vi "penningeject.vi"() -> ()   [LabVIEW 2014, in "Panels.lvlib"]
uses:
  Panels.lvlib
  CSlibraries-extern/DimLVEvent/DimIndicators/DimIndicators.lvlib
  CSCore/CSSystem/CoreLib/CoreLib.lvlib
  CSlibraries/UtilityLib/UtilityLib.valueStatus.ctl
  CSlibraries/UtilityLib/UtilityLib.lvlib
  CSlibraries-extern/DimLVEvent/LVDimInterface/LVDimInterface.lvlib
  Instance           1 20Saved   penningeject .vi
  CSlibraries-extern/DimLVEvent/DimIndicators/DimIndicators.numericType.ctl
  CSlibraries-extern/DimLVEvent/DimIndicators/DimIndicators.numericArrayType.ctl
  CSlibraries-extern/DimLVEvent/DimIndicators/DimIndicators.anyType.ctl
panel:
  in  "EjPenDT2":bool
  out "EjPenDT2_Mon":dbl=inf format="%.4f"
  in  "EjPenDT6":bool
  out "EjPenDT6_Mon":dbl=inf format="%.4f"
  in  "SetFileLocation_Data":T1={"data"="NOLINK", "no link"=TRUE, "quality"=-1, "timeStamp"=0.0}
  in  "SetFileLocation":path=path "\\\\intranet\\Files/projects/lebit/Data Exchange/data/PenningEjectControl"
  in  "EjPenDT3":bool
  in  "EjPenDT4":bool
  in  "EjPenDT1":bool
  out "EjPenDT4_Mon":dbl=inf format="%.4f"
  out "EjPenDT3_Mon":dbl=inf format="%.4f"
  out "i ref out":refnum<vi>
  in  "Last Loaded File_Data":T1={"data"="NOLINK", "no link"=TRUE, "quality"=-1, "timeStamp"=0.0}
  out "FileUpToDate":bool=TRUE caption="Parameter Changed"
  in  "Close All Panels":bool
  in  "EjPenDT2_SetValueInfoData":T2={"data"=[], "no link"=TRUE, "quality"=-1, "timeStamp"=0.0}
  in  "EjPenDT3_SetValueInfoData":T2={"data"=[], "no link"=TRUE, "quality"=-1, "timeStamp"=0.0}
  in  "EjPenDT4_SetValueInfoData":T2={"data"=[], "no link"=TRUE, "quality"=-1, "timeStamp"=0.0}
  in  "EjPenDT6_SetValueInfoData":T2={"data"=[], "no link"=TRUE, "quality"=-1, "timeStamp"=0.0}
  in  "EjPenDT1_SetValueInfoData":T2={"data"=[], "no link"=TRUE, "quality"=-1, "timeStamp"=0.0}
  in  "EjPenDT1_SetData":T2={"data"=[], "no link"=TRUE, "quality"=-1, "timeStamp"=0.0}
  in  "EjPenDT6_SetData":T2={"data"=[], "no link"=TRUE, "quality"=-1, "timeStamp"=0.0}
  in  "EjPenDT4_SetData":T2={"data"=[], "no link"=TRUE, "quality"=-1, "timeStamp"=0.0}
  in  "EjPenDT3_SetData":T2={"data"=[], "no link"=TRUE, "quality"=-1, "timeStamp"=0.0}
  in  "EjPenDT2_SetData":T2={"data"=[], "no link"=TRUE, "quality"=-1, "timeStamp"=0.0}
  out "Last Loaded File":string
  in  "EjPenDT6_MonData":T3={"data"=inf, "no link"=TRUE, "quality"=-1, "timeStamp"=0.0}
  in  "EjPenDT4_MonData":T3={"data"=inf, "no link"=TRUE, "quality"=-1, "timeStamp"=0.0}
  in  "EjPenDT3_MonData":T3={"data"=inf, "no link"=TRUE, "quality"=-1, "timeStamp"=0.0}
  in  "EjPenDT2_MonData":T3={"data"=inf, "no link"=TRUE, "quality"=-1, "timeStamp"=0.0}
  in  "EjPenDT1_MonData":T3={"data"=inf, "no link"=TRUE, "quality"=-1, "timeStamp"=0.0}
  out "EjPenDT1_Mon":dbl=inf format="%.4f"
  out "EjPenDT5_Mon":dbl=inf format="%.4f"
  # "Parameter changed, data file is no longer up-to-date."
  # "EJPenDT5"
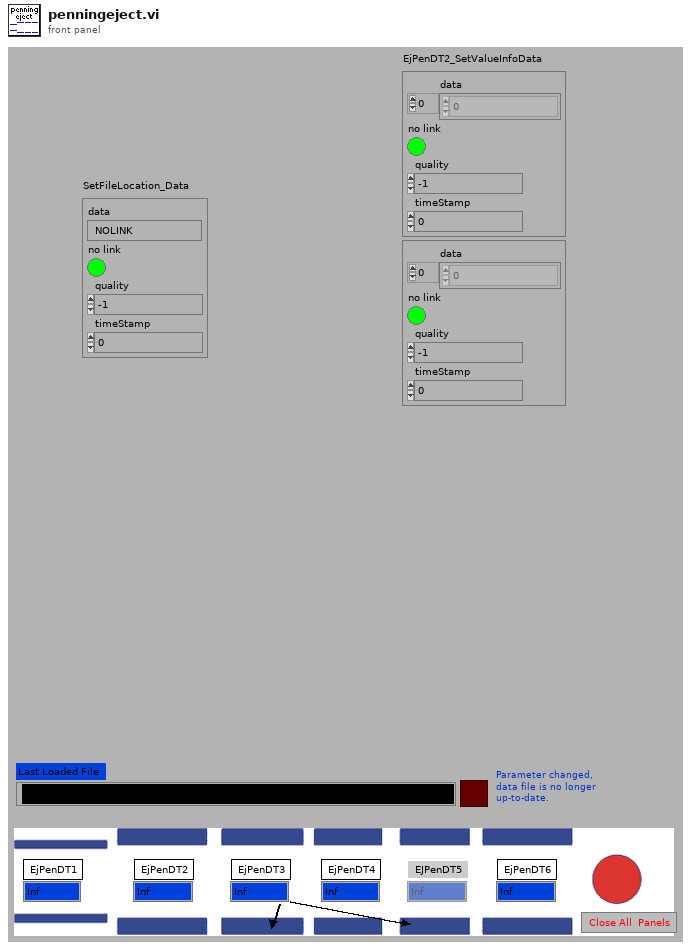
[diagram p1: front panel]
types:
  T1 = typedef "DimIndicators.lvlib/DimIndicators.anyType.ctl" = cluster{"data":string, "no link":bool, "quality":i32, "timeStamp":dbl}
  T2 = typedef "DimIndicators.lvlib/DimIndicators.numericArrayType.ctl" = cluster{"data":dbl[], "no link":bool, "quality":i32, "timeStamp":dbl}
  T3 = typedef "DimIndicators.lvlib/DimIndicators.numericType.ctl" = cluster{"data":dbl, "no link":bool, "quality":i32, "timeStamp":dbl}
  T4 = typedef "UtilityLib.lvlib/UtilityLib.valueStatus.ctl" = enum16{"no info available", "stand by/off", "on", "warning", "alarm/malfunction", "not implemented", "user action required", "important information", "system default", "control default", "indicator default", "button default"}
  T5 = cluster{"data":string, "no link":bool, "quality":i32, "timeStamp":dbl}
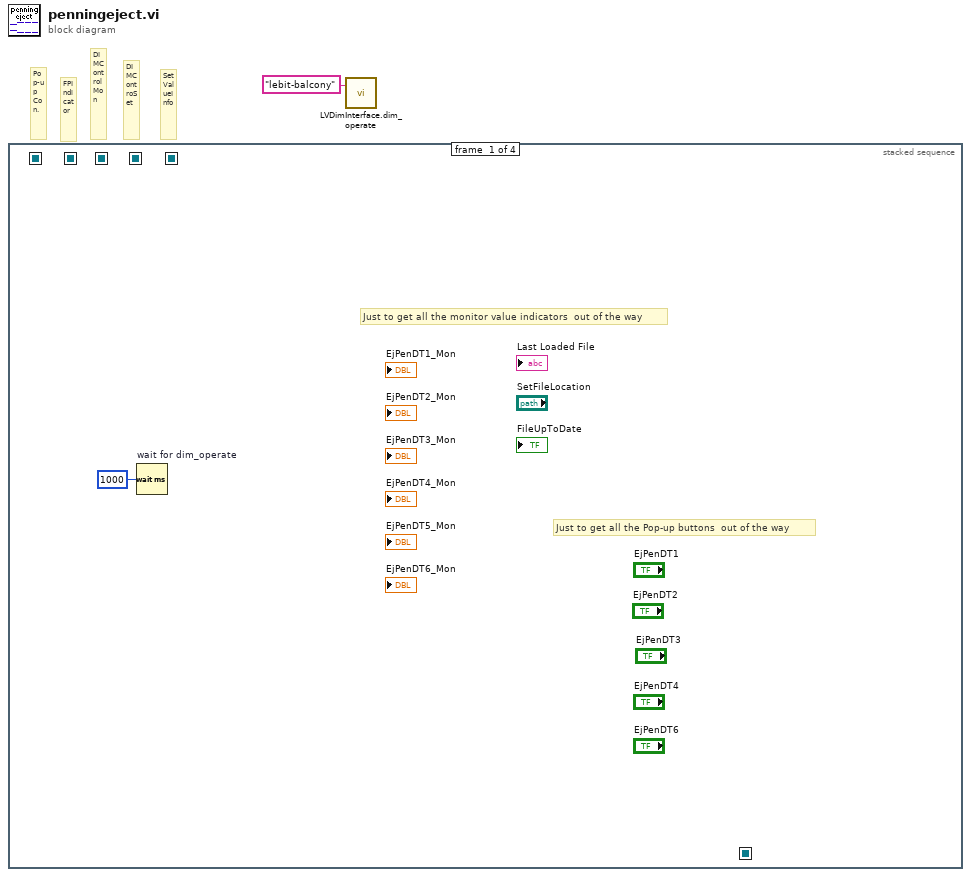
[diagram p0: block diagram]
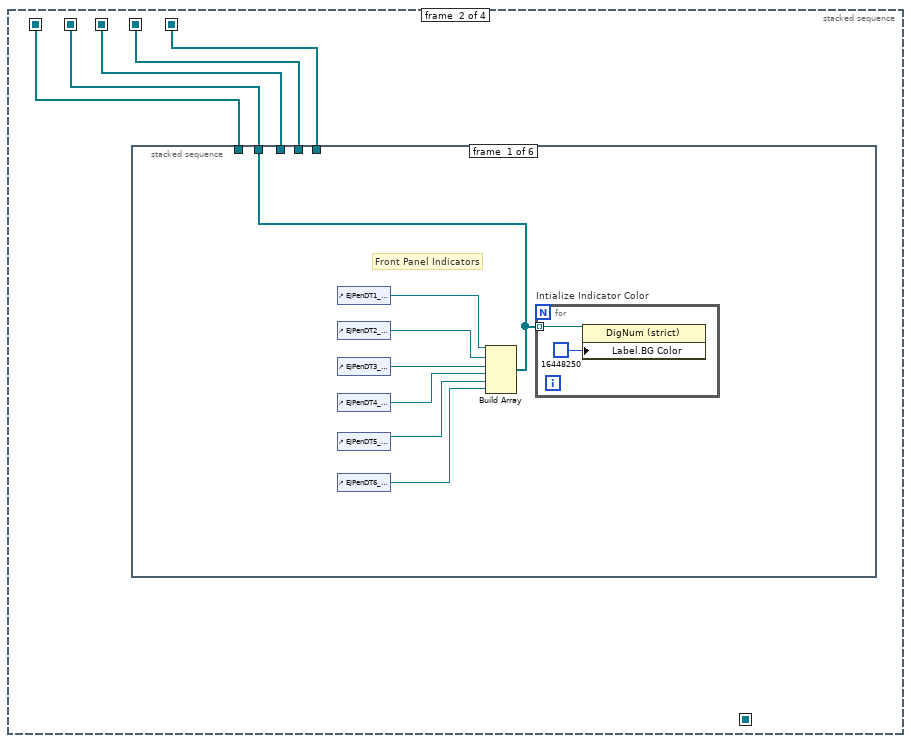
[diagram p2: hidden frame]
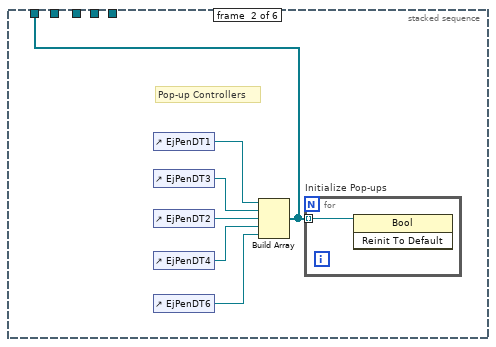
[diagram p3: hidden frame]
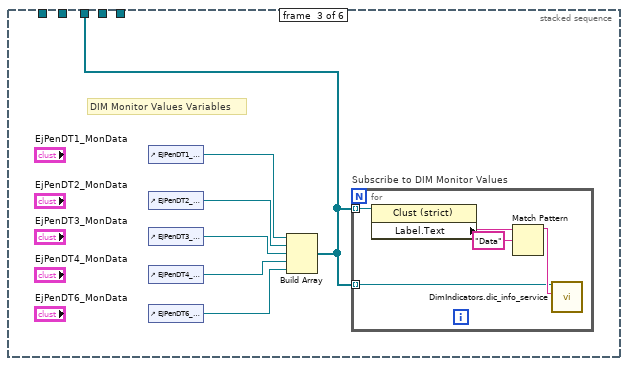
[diagram p4: hidden frame]
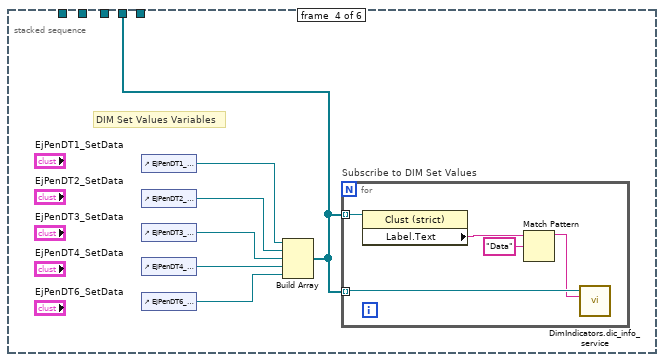
[diagram p5: hidden frame]
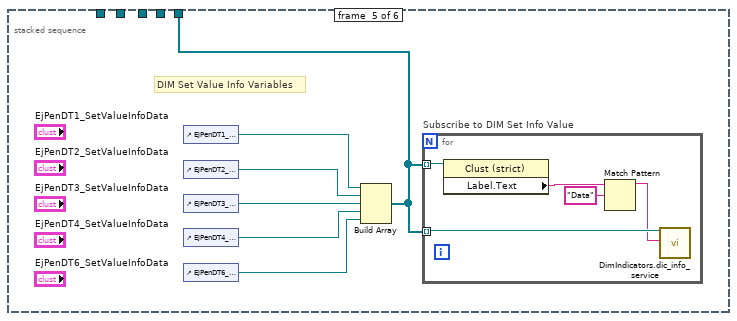
[diagram p6: hidden frame]
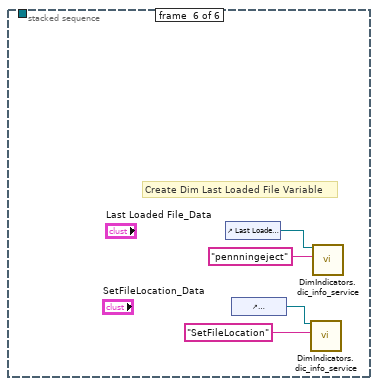
[diagram p7: hidden frame]
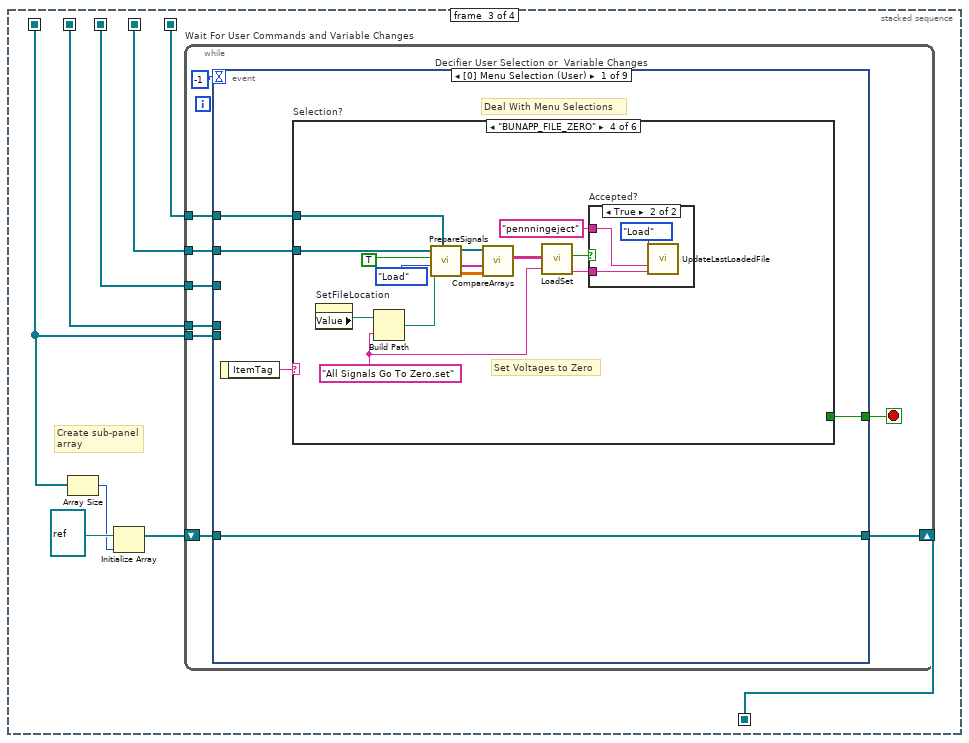
[diagram p8: hidden frame]
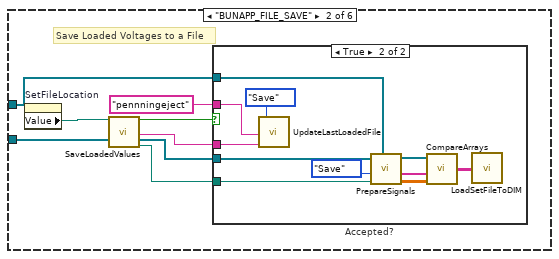
[diagram p10: hidden frame]
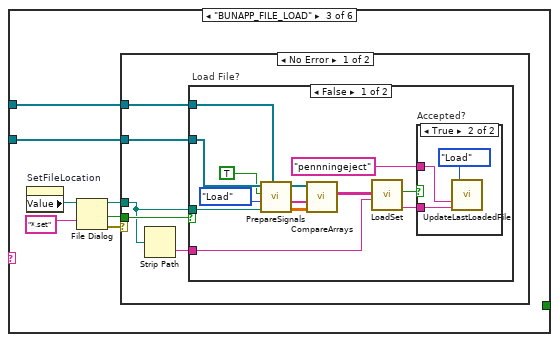
[diagram p12: hidden frame]
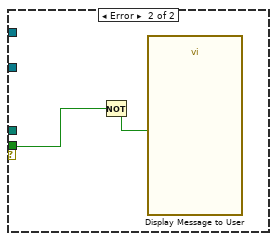
[diagram p15: hidden frame]
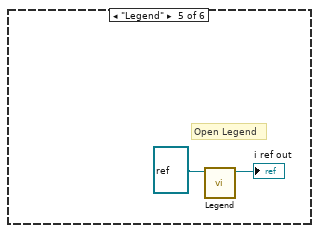
[diagram p17: hidden frame]
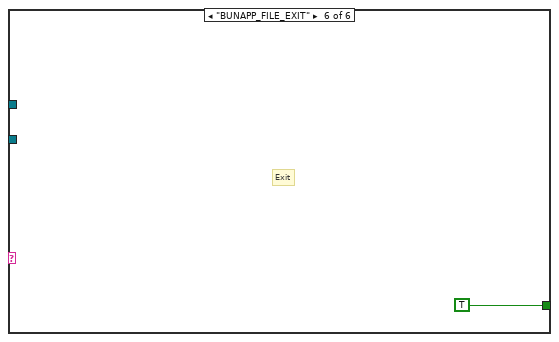
[diagram p18: hidden frame]
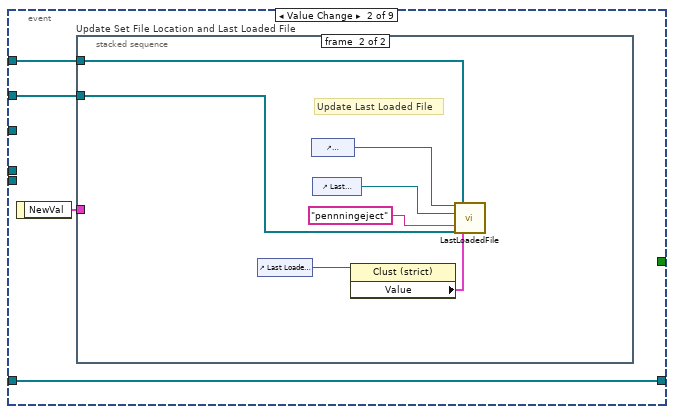
[diagram p19: hidden frame]
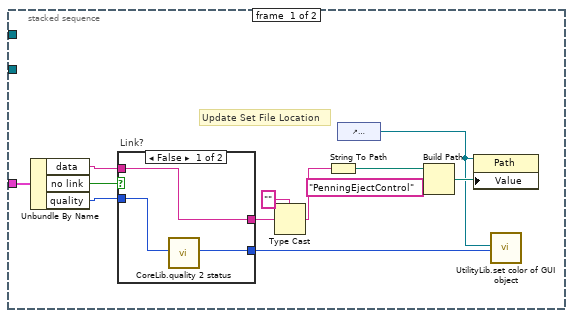
[diagram p20: hidden frame]
diagram:
  # "Pop-up Con."
  # "SetValueInfo"
  # "DIMControSet"
  # "DIMControlMon"
  # "FPIndicator"
  n1 = stacked-sequence {
    seq-local: [_ w7 _ _] -> [_ _ w66 _]
    seq-local: [_ w5 _ _] -> [_ _ w69 w265]
    seq-local: [_ _ w64 _] -> [_ _ _ w264]
    seq-local: [_ w4 _ _] -> [_ _ w63 w266]
    seq-local: [_ w3 _ _] -> [_ _ w62 w267]
    seq-local: [_ w6 _ _] -> [_ _ w61 _]
    frame #0 {
      # "Just to get all the Pop-up buttons  out of the way"
      # "Just to get all the monitor value indicators  out of the way"
      n2 = Wait (ms) "wait for dim_operate"(milliseconds to wait=u32 1000) -> ()  [unwired: 1 out]
    }
    frame #1 {
      # "Arrange references to all monitor-value related buttons into an array."
      n3 = stacked-sequence {
        tunnel: [w12 _ _ _ _ _] -> w7
        tunnel: [_ w19 _ _ _ _] -> w6
        tunnel: [_ _ w24 _ _ _] -> w5
        tunnel: [_ _ _ w35 _ _] -> w4
        tunnel: [_ _ _ _ w46 _] -> w3
        frame #0 {
          # "Front Panel Indicators"
          n4 = control-ref of="EjPenDT1_Mon"() -> (w11:refnum<vi>)
          n5 = control-ref of="EjPenDT2_Mon"() -> (w8:refnum<vi>)
          n6 = control-ref of="EjPenDT3_Mon"() -> (w10:refnum<vi>)
          n7 = control-ref of="EjPenDT4_Mon"() -> (w13:refnum<vi>)
          n8 = control-ref of="EjPenDT5_Mon"() -> (w14:refnum<vi>)
          n9 = control-ref of="EjPenDT6_Mon"() -> (w9:refnum<vi>)
          n10 = Build Array(w11, w8, w10, w13, w14, w9) -> (w12:refnum<vi>[])
          n11 = for "Intialize Indicator Color" {
            tunnel: w12 -> [w16] mode=indexing
            n12 = property class="DigNum (strict)"(reference=w16, "Label.BG Color"=u32 16448250 ("Color Box")) -> ()  [unwired: 1 in, 2 out]
          }
        }
        frame #1 {
          # "Pop-up Controllers"
          n13 = control-ref of="EjPenDT1"() -> (w22:refnum<vi>)
          n14 = control-ref of="EjPenDT3"() -> (w21:refnum<vi>)
          n15 = control-ref of="EjPenDT2"() -> (w18:refnum<vi>)
          n16 = control-ref of="EjPenDT4"() -> (w20:refnum<vi>)
          n17 = control-ref of="EjPenDT6"() -> (w17:refnum<vi>)
          n18 = Build Array(w22, w21, w18, w20, w17) -> (w19:refnum<vi>[])
          n19 = for "Initialize Pop-ups" {
            tunnel: w19 -> [w23] mode=indexing
            n20 = invoke class="Bool" method="Reinit To Default"(reference=w23) -> ()  [unwired: 2 in, 3 out]
          }
        }
        frame #2 {
          # "DIM Monitor Values Variables"
          n21 = control-ref of="EjPenDT1_MonData"() -> (w29:refnum<vi>)
          n22 = control-ref of="EjPenDT2_MonData"() -> (w28:refnum<vi>)
          n23 = control-ref of="EjPenDT3_MonData"() -> (w27:refnum<vi>)
          n24 = control-ref of="EjPenDT4_MonData"() -> (w26:refnum<vi>)
          n25 = control-ref of="EjPenDT6_MonData"() -> (w25:refnum<vi>)
          n26 = Build Array(w29, w28, w27, w26, w25) -> (w24:refnum<vi>[])
          n27 = for "Subscribe to DIM Monitor Values" {
            tunnel: w24 -> [w31] mode=indexing
            tunnel: w24 -> [w30] mode=indexing
            n28 = property class="Clust (strict)"(reference=w30) -> ("Label.Text"=w33:string)  [unwired: 1 in, 2 out]
            n29 = Match Pattern(string=w33, regular expression="Data") -> (before substring=w32:string)  [unwired: 1 in, 3 out]
            n30 = call "DimIndicators.dic_info_service.vi"("controlRef"=w31, "serviceName"=w32) -> ()  [unwired: 16 in, 2 out]
          }
        }
        frame #3 {
          # "DIM Set Values Variables"
          n31 = control-ref of="EjPenDT1_SetData"() -> (w40:refnum<vi>)
          n32 = control-ref of="EjPenDT2_SetData"() -> (w39:refnum<vi>)
          n33 = control-ref of="EjPenDT3_SetData"() -> (w38:refnum<vi>)
          n34 = control-ref of="EjPenDT4_SetData"() -> (w37:refnum<vi>)
          n35 = control-ref of="EjPenDT6_SetData"() -> (w36:refnum<vi>)
          n36 = Build Array(w40, w39, w38, w37, w36) -> (w35:refnum<vi>[])
          n37 = for "Subscribe to DIM Set Values" {
            tunnel: w35 -> [w41] mode=indexing
            tunnel: w35 -> [w45] mode=indexing
            n38 = property class="Clust (strict)"(reference=w41) -> ("Label.Text"=w44:string)  [unwired: 1 in, 2 out]
            n39 = Match Pattern(string=w44, regular expression="Data") -> (before substring=w42:string)  [unwired: 1 in, 3 out]
            n40 = call "DimIndicators.dic_info_service.vi"("controlRef"=w45, "serviceName"=w42) -> ()  [unwired: 16 in, 2 out]
          }
        }
        frame #4 {
          # "DIM Set Value Info Variables"
          n41 = control-ref of="EjPenDT1_SetValueInfoData"() -> (w51:refnum<vi>)
          n42 = control-ref of="EjPenDT2_SetValueInfoData"() -> (w50:refnum<vi>)
          n43 = control-ref of="EjPenDT3_SetValueInfoData"() -> (w49:refnum<vi>)
          n44 = control-ref of="EjPenDT4_SetValueInfoData"() -> (w48:refnum<vi>)
          n45 = control-ref of="EjPenDT6_SetValueInfoData"() -> (w47:refnum<vi>)
          n46 = Build Array(w51, w50, w49, w48, w47) -> (w46:refnum<vi>[])
          n47 = for "Subscribe to DIM Set Info Value" {
            tunnel: w46 -> [w52] mode=indexing
            tunnel: w46 -> [w56] mode=indexing
            n48 = property class="Clust (strict)"(reference=w52) -> ("Label.Text"=w55:string)  [unwired: 1 in, 2 out]
            n49 = Match Pattern(string=w55, regular expression="Data") -> (before substring=w53:string)  [unwired: 1 in, 3 out]
            n50 = call "DimIndicators.dic_info_service.vi"("controlRef"=w56, "serviceName"=w53) -> ()  [unwired: 16 in, 2 out]
          }
        }
        frame #5 {
          # "Create Dim Last Loaded File Variable"
          n51 = control-ref of="Last Loaded File_Data"() -> (w59:refnum<vi>)
          n52 = control-ref of="SetFileLocation_Data"() -> (w57:refnum<vi>)
          n53 = call "DimIndicators.dic_info_service.vi"("controlRef"=w57, "serviceName"="SetFileLocation" ("string")) -> ()  [unwired: 16 in, 2 out]
          n54 = call "DimIndicators.dic_info_service.vi"("controlRef"=w59, "serviceName"="pennningeject" ("string")) -> ()  [unwired: 16 in, 2 out]
        }
      }
    }
    frame #2 {
      # "Create sub-panel\narray"
      n55 = Array Size(array=w61) -> (size(s)=w65:i32)
      n56 = Initialize Array(refnum<vi> refnum ("vi reference"), w65) -> (w68:refnum<vi>[])
      n57 = while "Wait For User Commands and Variable Changes" {
        tunnel: w69 -> [w77]
        tunnel: w66 -> [w76]
        shift-right: [w74] -> w64
        shift-left: w68 -> [w75]
        tunnel: w63 -> [w73]
        tunnel: w62 -> [w72]
        tunnel: w61 -> [w70]
        stop <- w78 stop-if-true
        n58 = event "Decifier User Selection or  Variable Changes" shown="[0] Menu Selection (User)" {
          selector: _ -> [_ _ _ _ _ _ _ _ _]
          dyn-events: _ -> [_ _ _ _ _ _ _ _ _]
          timeout: -1 -> [_ _ _ _ _ _ _ _ _]
          tunnel: [w80 _ _ _ _ _ _ _ TRUE ("stop")] -> w78
          tunnel: w77 -> [_ _ _ _ _ _ _ _ w240]
          tunnel: w76 -> [_ _ _ w190 _ _ _ _ _]
          tunnel: w75 -> [w83 w155 w187 w189 w217 w225 w232 w238 w239]
          tunnel: [w83 w155 w187 w189 w217 w223 w230 w238 _] -> w74
          tunnel: w73 -> [w81 w154 w184 _ w214 _ _ _ w241]
          tunnel: w72 -> [w79 w153 w181 _ _ _ _ _ w242]
          tunnel: w70 -> [_ _ _ _ _ w219 _ _ _]
          event Menu Selection (User) {
            # "Deal With Menu Selections"
            n59 = event-data() -> ("ItemTag"=w82:string)  [unwired: 1 in]
            n60 = case "Selection?" shown="\"BUNAPP_FILE_ZERO\"" w82 {
              tunnel: w81 -> [_ w88 w108 w146 _ _]
              tunnel: [_ _ _ _ _ TRUE ("stop")] -> w80
              tunnel: w79 -> [_ w84 w103 w133 _ _]
              frame "False", Default {
              }
              frame "BUNAPP_FILE_SAVE" {
                # "Save Loaded Voltages to a File"
                n61 = property on="SetFileLocation" class="Path"() -> ("Value"=w89:path)  [unwired: 2 in, 2 out]
                n62 = call "SaveLoadedValues.vi"("Panel Location?"=w89, "DIMControlSet in"=w88) -> ("File Saved?"=w90:bool, "File Name"=w87:string, "DIMControlSet out"=w85:refnum<vi>[], "Path"=w86:path)  [unwired: 14 in]
                n63 = case "Accepted?" shown="True" w90 {
                  tunnel: w87 -> [_ w100]
                  tunnel: "pennningeject" ("string") -> [_ w102]
                  tunnel: w85 -> [_ w101]
                  tunnel: w86 -> [_ w99]
                  tunnel: w84 -> [_ w93]
                  frame False {
                  }
                  frame True {
                    n64 = call "UpdateLastLoadedFile.vi"("LoadOrSave"=enum16{"Load", "Save"}."Save", "GUIName"=w102, "FileNameIn"=w100) -> ()  [unwired: 13 in]
                    n65 = call "PrepareSignals.vi"("SetValueInfo in"=w93, "setfile path"=w99, "Enum"=enum16{"Save", "Load"}."Save", "DIMControSet in"=w101) -> ("indexed loaded Array"=w97:dbl[][], "Name Array"=w98:string[], "DIMControSet out"=w96:refnum<vi>[])  [unwired: 5 in]
                    n66 = call "CompareArrays.vi"("indexed loaded Array"=w97, "Name Array"=w98, "DIMControSet"=w96) -> ("Table for loading values"=w95:string[][])  [unwired: 4 in]
                    n67 = call "LoadSetFileToDIM.vi"("output array"=w95) -> ()  [unwired: 2 in]
                  }
                }
              }
              frame "BUNAPP_FILE_LOAD" {
                # "Promt User For File to Load"
                n68 = property on="SetFileLocation" class="Path"() -> ("Value"=w105:path)  [unwired: 2 in, 2 out]
                n69 = File Dialog(6:"*.set" ("pattern (all files)"), 11:w105) -> (0:w104:errorcluster, 1:w109:bool, 3:w106:path)  [unwired: 5 in, 1 out]
                n70 = case shown="No Error" w104 {
                  tunnel: w109 -> [w114 w131]
                  tunnel: w108 -> [w113 _]
                  tunnel: w106 -> [w111 _]
                  tunnel: w103 -> [w110 _]
                  frame No Error {
                    n71 = Strip Path(path=w111) -> (name=w112:string)  [unwired: 1 out]
                    n72 = case "Load File?" shown="False" w114 {
                      tunnel: w113 -> [w127 _]
                      tunnel: w112 -> [w121 _]
                      tunnel: w111 -> [w122 _]
                      tunnel: w110 -> [w115 _]
                      frame False {
                        n73 = call "PrepareSignals.vi"("SetValueInfo in"=w115, "setfile path"=w122, "Enum"=enum16{"Save", "Load"}."Load", "Display Message to \nUser"=TRUE ("Display Message to \nUser"), "DIMControSet in"=w127) -> ("indexed loaded Array"=w125:dbl[][], "Name Array"=w124:string[], "DIMControSet out"=w126:refnum<vi>[])  [unwired: 4 in]
                        n74 = call "CompareArrays.vi"("indexed loaded Array"=w125, "Name Array"=w124, "DIMControSet"=w126) -> ("Table for loading values"=w123:string[][])  [unwired: 4 in]
                        n75 = call "LoadSet.vi"("File Name In"=w121, "output array"=w123) -> ("File Name out"=w120:string, "Accepted"=w119:bool)  [unwired: 8 in]
                        n76 = case "Accepted?" shown="True" w119 {
                          tunnel: w120 -> [_ w130]
                          tunnel: "pennningeject" ("string") -> [_ w129]
                          frame False {
                          }
                          frame True {
                            n77 = call "UpdateLastLoadedFile.vi"("LoadOrSave"=enum16{"Load", "Save"}."Load", "GUIName"=w129, "FileNameIn"=w130) -> ()  [unwired: 13 in]
                          }
                        }
                      }
                      frame True {
                      }
                    }
                  }
                  frame Error {
                    n78 = Not(x=w131) -> (.not. x?=w132:bool)
                    n79 = call "Display Message to User"("Enable"=w132) -> ()  [unwired: 9 in, 2 out]
                  }
                }
              }
              frame "BUNAPP_FILE_ZERO" {
                w137 = "All Signals Go To Zero.set" ("File Name")
                # "Set Voltages to Zero"
                n80 = property on="SetFileLocation" class="Path"() -> ("Value"=w135:path)  [unwired: 2 in, 2 out]
                n81 = Build Path(base path=w135, name or relative path=w137) -> (appended path=w136:path)
                n82 = call "PrepareSignals.vi"("SetValueInfo in"=w133, "setfile path"=w136, "Enum"=enum16{"Save", "Load"}."Load", "Display Message to \nUser"=TRUE ("Display Message to \nUser"), "DIMControSet in"=w146) -> ("indexed loaded Array"=w144:dbl[][], "Name Array"=w143:string[], "DIMControSet out"=w145:refnum<vi>[])  [unwired: 4 in]
                n83 = call "CompareArrays.vi"("indexed loaded Array"=w144, "Name Array"=w143, "DIMControSet"=w145) -> ("Table for loading values"=w142:string[][])  [unwired: 4 in]
                n84 = call "LoadSet.vi"("File Name In"=w137, "output array"=w142) -> ("File Name out"=w140:string, "Accepted"=w141:bool)  [unwired: 8 in]
                n85 = case "Accepted?" shown="True" w141 {
                  tunnel: w140 -> [_ w149]
                  tunnel: "pennningeject" ("string") -> [_ w148]
                  frame False {
                  }
                  frame True {
                    n86 = call "UpdateLastLoadedFile.vi"("LoadOrSave"=enum16{"Load", "Save"}."Load", "GUIName"=w148, "FileNameIn"=w149) -> ()  [unwired: 13 in]
                  }
                }
              }
              frame "Legend" {
                # "Open Legend"
                n87 = call "Legend.vi"("i ref in"=refnum<vi> refnum) -> ("i ref out"=→"i ref out":refnum<vi>)  [unwired: 10 in]
              }
              frame "BUNAPP_FILE_EXIT" {
                # "Exit"
              }
            }
          }
          event Value Change {
            n88 = event-data() -> ("NewVal"=w156:T1)  [unwired: 1 in]
            n89 = stacked-sequence "Update Set File Location and Last Loaded File" {
              tunnel: w156 -> [w158 _]
              tunnel: w154 -> [_ w178]
              tunnel: w153 -> [_ w174]
              frame #0 {
                # "Update Set File Location"
                n90 = Unbundle By Name(w158) -> ("data"=w167:string, "no link"=w166:bool, "quality"=w165:i32)
                n91 = case "Link?" shown="False" w166 {
                  tunnel: w165 -> [w171 _]
                  tunnel: [w170 UtilityLib.valueStatus."no info available" ("valueStatus")] -> w168
                  tunnel: w167 -> [w169 _]
                  tunnel: [w169 w172] -> w163
                  frame False {
                    n92 = call "CoreLib.quality 2 status.vi"("quality"=w171) -> ("valueStatus"=w170:T4)  [unwired: 18 in]
                  }
                  frame True {
                    n93 = call "EmptyString.vi"() -> ("String"=w172:string)
                  }
                }
                n94 = Type Cast(type="" ("regular expression"), x=w163) -> (*(type *) &x=w162:string)
                n95 = String To Path(string=w162) -> (path=w159:path)
                n96 = control-ref of="SetFileLocation"() -> (w157:refnum<vi>)
                n97 = Build Path(base path=w159, name or relative path="PenningEjectControl") -> (appended path=w160:path)
                n98 = property class="Path"(reference=w157, "Value"=w160) -> ()  [unwired: 1 in, 2 out]
                n99 = call "UtilityLib.set color of GUI object.vi"("GUI object Ref"=w157, "valueStatus"=w168) -> ()  [unwired: 17 in, 1 out]
              }
              frame #1 {
                # "Update Last Loaded File"
                n100 = control-ref of="Last Loaded File_Data"() -> (w175:refnum<vi>)
                n101 = control-ref of="SetFileLocation"() -> (w177:refnum<vi>)
                n102 = control-ref of="Last Loaded File"() -> (w176:refnum<vi>)
                n103 = property class="Clust (strict)"(reference=w175) -> ("Value"=w180:T5)  [unwired: 1 in, 2 out]
                n104 = call "LastLoadedFile.vi"("SetFileLocation"=w177, "Last Loaded File"=w176, "GUIName"="pennningeject" ("string"), "DIMControSet in"=w178, "SetValueInfo in"=w174, "NewVal"=w180) -> ()  [unwired: 14 in]
              }
            }
          }
          event Value Change {
            # "Update Last Loaded File"
            n105 = event-data() -> ("NewVal"=w186:T1)  [unwired: 1 in]
            n106 = control-ref of="SetFileLocation"() -> (w183:refnum<vi>)
            n107 = control-ref of="Last Loaded File"() -> (w182:refnum<vi>)
            n108 = call "LastLoadedFile.vi"("SetFileLocation"=w183, "Last Loaded File"=w182, "GUIName"="pennningeject" ("string"), "DIMControSet in"=w184, "SetValueInfo in"=w181, "NewVal"=w186) -> ()  [unwired: 14 in]
          }
          event Value Change {
            n109 = event-data() -> ("CtlRef"=w188:refnum<vi>, "NewVal"=w191:T3)  [unwired: 1 in, 4 out]
            n110 = for "Check if Indicator Exists for the Monitor Value?" {
              tunnel: w191 -> [w200]
              tunnel: w190 -> [w197] mode=indexing
              tunnel: w188 -> [w196]
              # "Updating a Monitor Value"
              n111 = property class="DigNum (strict)"(reference=w197) -> (reference out=w192:refnum<vi>, "Label.Text"=w194:string)  [unwired: 1 in, 1 out]
              n112 = property class="Clust (strict)"(reference=w196) -> ("Label.Text"=w198:string)  [unwired: 1 in, 2 out]
              n113 = Match Pattern(string=w198, regular expression="Data") -> (before substring=w193:string)  [unwired: 1 in, 3 out]
              n114 = Equal?(x=w194, y=w193) -> (x = y?=w195:bool)
              n115 = case "Indicator exists?" shown="True" w195 {
                tunnel: w200 -> [w207 _]
                tunnel: w192 -> [w201 _]
                frame True {
                  n116 = Unbundle By Name(w207) -> ("data"=w203:dbl, "no link"=w204:bool, "quality"=w206:i32)
                  n117 = case shown="True" w204 {
                    tunnel: w206 -> [w210 _]
                    tunnel: [w209 UtilityLib.valueStatus."no info available" ("valueStatus")] -> w205
                    tunnel: w203 -> [w208 _]
                    tunnel: [w208 inf] -> w202
                    frame False {
                      n118 = call "CoreLib.quality 2 status.vi"("quality"=w210) -> ("valueStatus"=w209:T4)  [unwired: 18 in]
                    }
                    frame True {
                    }
                  }
                  n119 = property class="DigNum (strict)"(reference=w201, "Value"=w202) -> ()  [unwired: 1 in, 2 out]
                  n120 = call "TextColor.vi"("valueStatus"=w205, "reference"=w201) -> ()  [unwired: 10 in]
                }
                frame False {
                }
              }
            }
          }
          event Value Change {
            n121 = event-data() -> ("CtlRef"=w215:refnum<vi>)  [unwired: 1 in, 5 out]
            n122 = property on="FileUpToDate" class="Bool (strict)"() -> ("Value"=w213:bool)  [unwired: 2 in, 2 out]
            n123 = call "FileUpToDate.vi"("FileUpToDate in"=w213, "DIMControSet out"=w214, "CtlRef"=w215) -> ("FileUpToDate out"=w216:bool)  [unwired: 16 in]
            n124 = property on="FileUpToDate" class="Bool (strict)"("Value"=w216) -> ()  [unwired: 2 in, 2 out]
          }
          event "EjPenDT1", "EjPenDT4", "EjPenDT3", "EjPenDT2", "EjPenDT6": Value Change {
            # "Find sub-panel index"
            # "opening or closing a sub-panel"
            n125 = event-data() -> ("CtlRef"=w218:refnum<vi>)  [unwired: 1 in, 3 out]
            n126 = Search 1D Array(1D array=w219, element=w218) -> (index of element=w224:i32)  [unwired: 1 in]
            n127 = Index Array(array=w225, index=w224) -> (element=w222:refnum<vi>)
            n128 = invoke class="Bool" method="Reinit To Default"(reference=w218) -> ()  [unwired: 2 in, 3 out]
            n129 = property class="VI"(reference=w222) -> ("Front Panel.Open"=w221:bool)  [unwired: 1 in, 2 out]
            n130 = case "Panel Already Open?" shown="False" w221 {
              tunnel: w218 -> [w226 _]
              tunnel: w222 -> [_ w229]
              tunnel: [w227 refnum<vi> refnum ("vi reference")] -> w220
              frame False {
                n131 = call "OpenPanel.vi"("CtlRef"=w226) -> ("vi reference"=w227:refnum<vi>)  [unwired: 2 in]
              }
              frame True {
                n132 = call "PanelClose.vi"("vi reference"=w229) -> ()
              }
            }
            n133 = Replace Array Subset(array=w225, new element=w220, index=w224) -> (w223:refnum<vi>[])
          }
          event "Close All Panels": Value Change {
            n134 = event-data() -> ()  [unwired: 1 in, 6 out]
            n135 = case "Close Open Panels?" shown="True" "Close All Panels" {
              tunnel: w232 -> [w233 w235]
              tunnel: [w233 w234] -> w230
              frame False {
              }
              frame True {
                n136 = for "Close Open Panels" {
                  tunnel: w235 -> [w237] mode=indexing
                  tunnel: w235 -> [w236]
                  tunnel: [w236] -> w234
                  n137 = call "PanelClose.vi"("vi reference"=w237) -> ()
                }
              }
            }
          }
          event Timeout {
            # "Timeout"
            n138 = event-data() -> ()  [unwired: 1 in, 3 out]
          }
          event Panel Close? {
            n139 = event-data() -> ()  [unwired: 1 in, 4 out]
            n140 = stacked-sequence {
              tunnel: w242 -> [w248 _]
              tunnel: w241 -> [w247 _]
              tunnel: w240 -> [w246 _]
              tunnel: w239 -> [w249 _]
              frame #0 {
                # "Release DIM Services"
                n141 = for "Close Open Panels" {
                  tunnel: w249 -> [w259] mode=indexing
                  n142 = call "PanelClose.vi"("vi reference"=w259) -> ()
                }
                n143 = for "For Each Service" {
                  tunnel: w248 -> [w257] mode=indexing
                  n144 = Not A Number/Path/Refnum?(number/path/refnum=w257) -> (NaN/Path/Refnum?=w256:bool)
                  n145 = case "Not a Reference?" shown="False" w256 {
                    tunnel: w257 -> [w258 _]
                    frame False {
                      n146 = call "DimIndicators.dic_release_service.vi"("controlRef"=w258) -> ()  [unwired: 18 in, 1 out]
                    }
                    frame True {
                    }
                  }
                }
                n147 = for "For Each Service" {
                  tunnel: w247 -> [w254] mode=indexing
                  n148 = Not A Number/Path/Refnum?(number/path/refnum=w254) -> (NaN/Path/Refnum?=w253:bool)
                  n149 = case "Not a Reference?" shown="False" w253 {
                    tunnel: w254 -> [w255 _]
                    frame False {
                      n150 = call "DimIndicators.dic_release_service.vi"("controlRef"=w255) -> ()  [unwired: 18 in, 1 out]
                    }
                    frame True {
                    }
                  }
                }
                n151 = for "For Each Service" {
                  tunnel: w246 -> [w251] mode=indexing
                  n152 = Not A Number/Path/Refnum?(number/path/refnum=w251) -> (NaN/Path/Refnum?=w250:bool)
                  n153 = case "Not a Reference?" shown="False" w250 {
                    tunnel: w251 -> [w252 _]
                    frame False {
                      n154 = call "DimIndicators.dic_release_service.vi"("controlRef"=w252) -> ()  [unwired: 18 in, 1 out]
                    }
                    frame True {
                    }
                  }
                }
                n155 = control-ref of="Last Loaded File_Data"() -> (w245:refnum<vi>)
                n156 = control-ref of="SetFileLocation_Data"() -> (w244:refnum<vi>)
                n157 = call "DimIndicators.dic_release_service.vi"("controlRef"=w245) -> ()  [unwired: 18 in, 1 out]
                n158 = call "DimIndicators.dic_release_service.vi"("controlRef"=w244) -> ()  [unwired: 18 in, 1 out]
              }
              frame #1 {
                # "Close Front Panel"
                n159 = Current VI's Path() -> (path=w260:path)
                n160 = Open VI Reference(vi path=w260) -> (vi reference=w262:refnum<vi>, error out=w263:errorcluster)  [unwired: 5 in]
                n161 = property class="VI"(reference=w262, error in=w263, "Front Panel Window:Open"=FALSE) -> ()  [unwired: 2 out]
              }
            }
            n162 = event-data() -> ()  [unwired: 2 in, 1 out]
          }
        }
      }
    }
    frame #3 {
      n163 = stacked-sequence {
        tunnel: w264 -> [w273 _ _]
        tunnel: w266 -> [w271 _ _]
        tunnel: w267 -> [w272 _ _]
        tunnel: w265 -> [w270 _ _]
        frame #0 {
          # "Release DIM Services"
          n164 = control-ref of="Last Loaded File_Data"() -> (w269:refnum<vi>)
          n165 = control-ref of="SetFileLocation_Data"() -> (w268:refnum<vi>)
          n166 = call "DimIndicators.dic_release_service.vi"("controlRef"=w269) -> ()  [unwired: 18 in, 1 out]
          n167 = call "DimIndicators.dic_release_service.vi"("controlRef"=w268) -> ()  [unwired: 18 in, 1 out]
          n168 = for "For Each Service" {
            tunnel: w272 -> [w281] mode=indexing
            n169 = Not A Number/Path/Refnum?(number/path/refnum=w281) -> (NaN/Path/Refnum?=w280:bool)
            n170 = case "Not a Reference?" shown="False" w280 {
              tunnel: w281 -> [w282 _]
              frame False {
                n171 = call "DimIndicators.dic_release_service.vi"("controlRef"=w282) -> ()  [unwired: 18 in, 1 out]
              }
              frame True {
              }
            }
          }
          n172 = for "For Each Service" {
            tunnel: w271 -> [w278] mode=indexing
            n173 = Not A Number/Path/Refnum?(number/path/refnum=w278) -> (NaN/Path/Refnum?=w277:bool)
            n174 = case "Not a Reference?" shown="False" w277 {
              tunnel: w278 -> [w279 _]
              frame False {
                n175 = call "DimIndicators.dic_release_service.vi"("controlRef"=w279) -> ()  [unwired: 18 in, 1 out]
              }
              frame True {
              }
            }
          }
          n176 = for "For Each Service" {
            tunnel: w270 -> [w275] mode=indexing
            n177 = Not A Number/Path/Refnum?(number/path/refnum=w275) -> (NaN/Path/Refnum?=w274:bool)
            n178 = case "Not a Reference?" shown="False" w274 {
              tunnel: w275 -> [w276 _]
              frame False {
                n179 = call "DimIndicators.dic_release_service.vi"("controlRef"=w276) -> ()  [unwired: 18 in, 1 out]
              }
              frame True {
              }
            }
          }
          n180 = for "Close Open Panels" {
            tunnel: w273 -> [w283] mode=indexing
            n181 = call "PanelClose.vi"("vi reference"=w283) -> ()
          }
        }
        frame #1 {
          # "Close Front Panel"
          n182 = Current VI's Path() -> (path=w287:path)
          n183 = Open VI Reference(vi path=w287) -> (vi reference=w285:refnum<vi>, error out=w284:errorcluster)  [unwired: 5 in]
          n184 = property class="VI"(reference=w285, error in=w284, "Front Panel Window:Open"=FALSE) -> ()  [unwired: 2 out]
        }
        frame #2 {
          # "Stop Panel"
          n185 = Stop(stop? (T)=TRUE) -> ()
        }
      }
    }
  }
  n186 = call "LVDimInterface.dim_operate.vi"("DNSNode"="lebit-balcony" ("DNS node")) -> ()  [unwired: 19 in]
